vi "main.vi"() -> ()   [LabVIEW 2016]
uses:
  <vilib>/Instr/_visa.llb/VISA Configure Serial Port (Instr).vi
panel:
  out "强度图":dbl[][](graph)
  out "judge":i32=1
  out "Xloop":dbl
  out "判定":dbl
  out "幅频谱":dbl[](graph)
  out "时域谱":dbl[](graph)
  out "错误输出":errorcluster
  in  "启动":bool
  in  "开始扫描":bool
  in  "X归零":bool
  in  "Y归零":bool
  in  "Y":dbl
  in  "Y轴速度":dbl=3000.0
  in  "X轴速度":dbl=3000.0
  out "电机状态":bool
  out "error out":errorcluster caption="步进电机"
  in  "电机端口":refnum<visa-resource-name>="COM3"
  out "Yloop":dbl
  in  "X扫描范围":dbl
  in  "Y扫描范围":dbl=1.0
  out "Y序":i32
  in  "X":dbl
  out "Y(mm)":dbl
  out "x+y 2":dbl
  in  "Y步进":dbl=1.0
  in  "精度":dbl
  in  "电机急停":bool
  out "X（mm）":dbl
  out "x+y":dbl
  in  "X步进":dbl=1.0
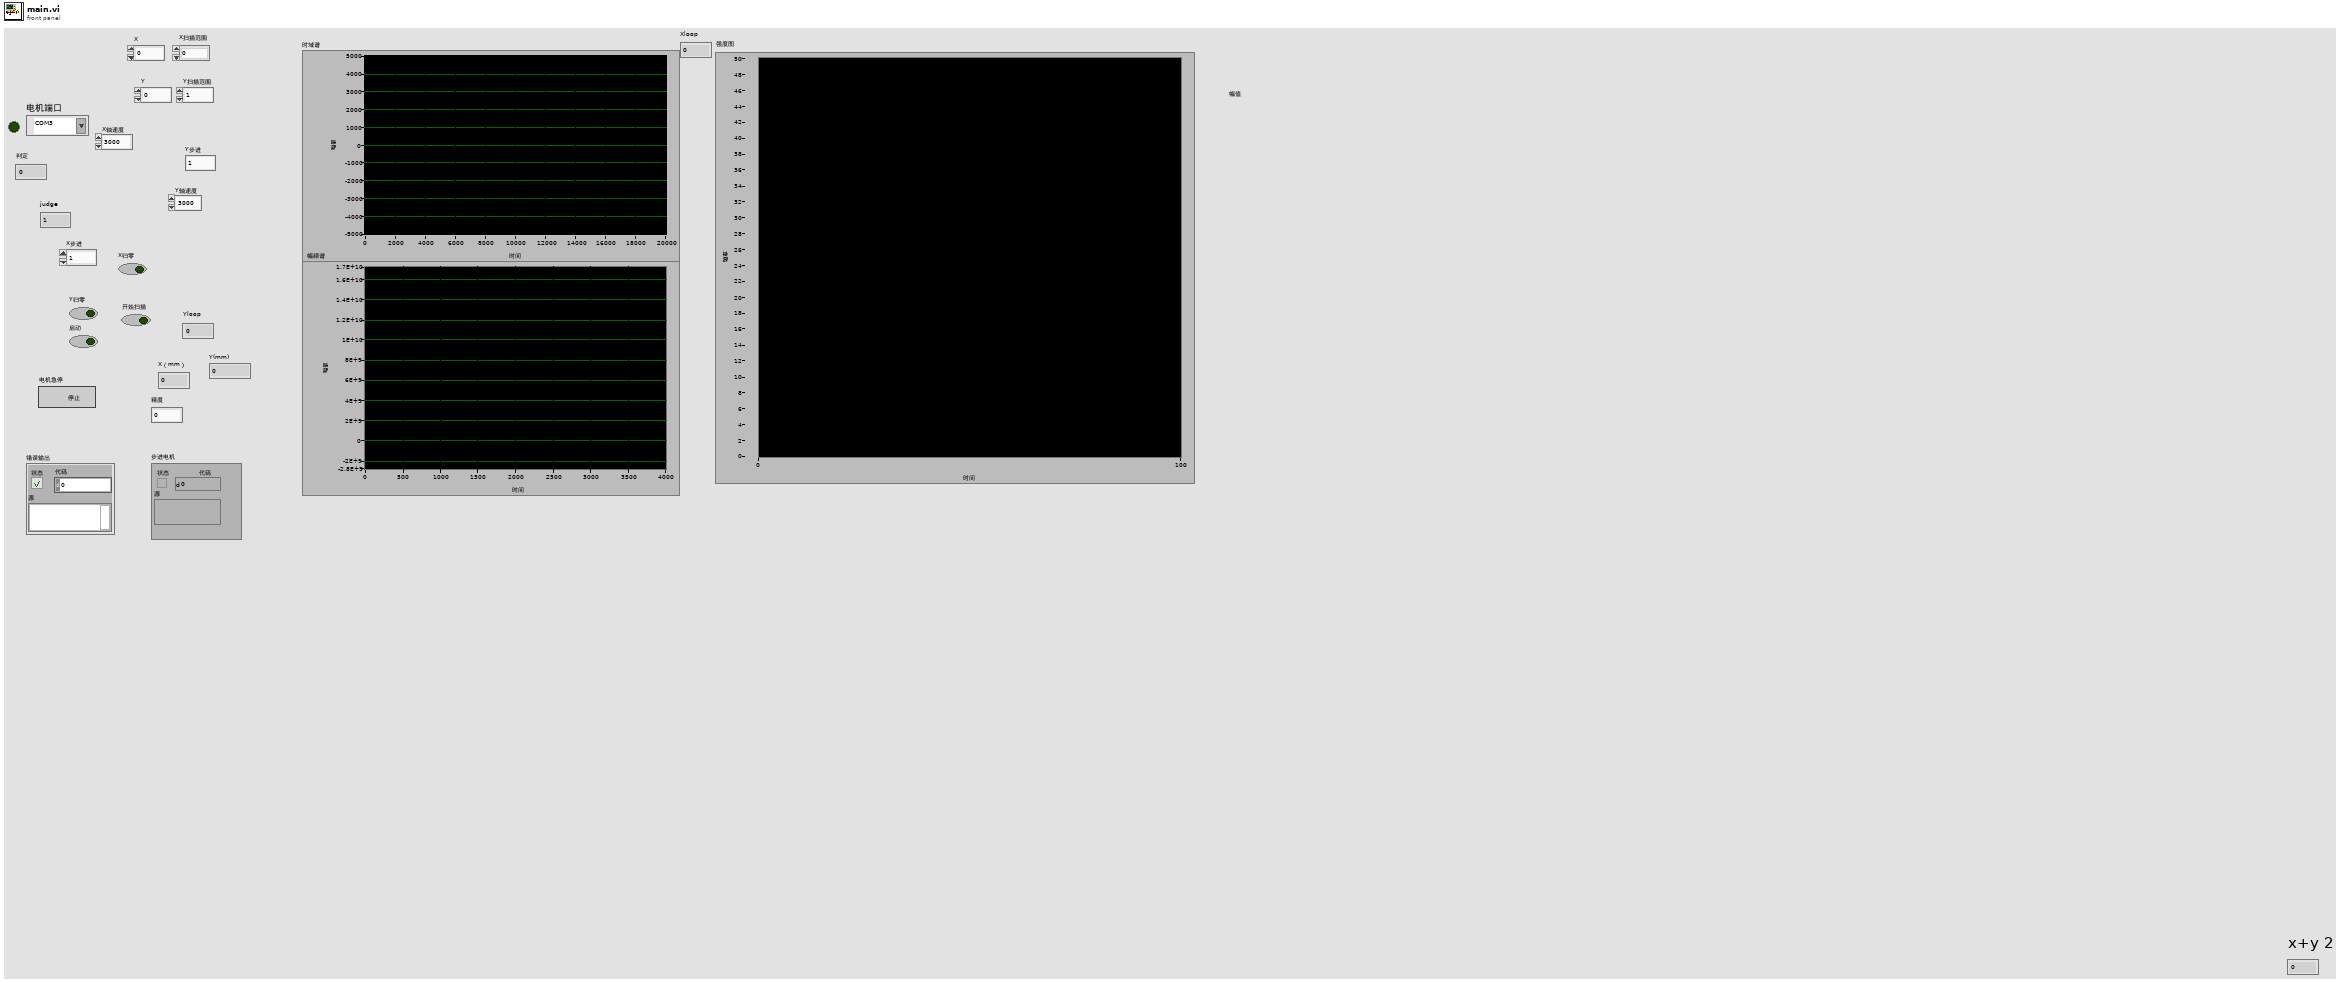
[diagram p1: front panel]
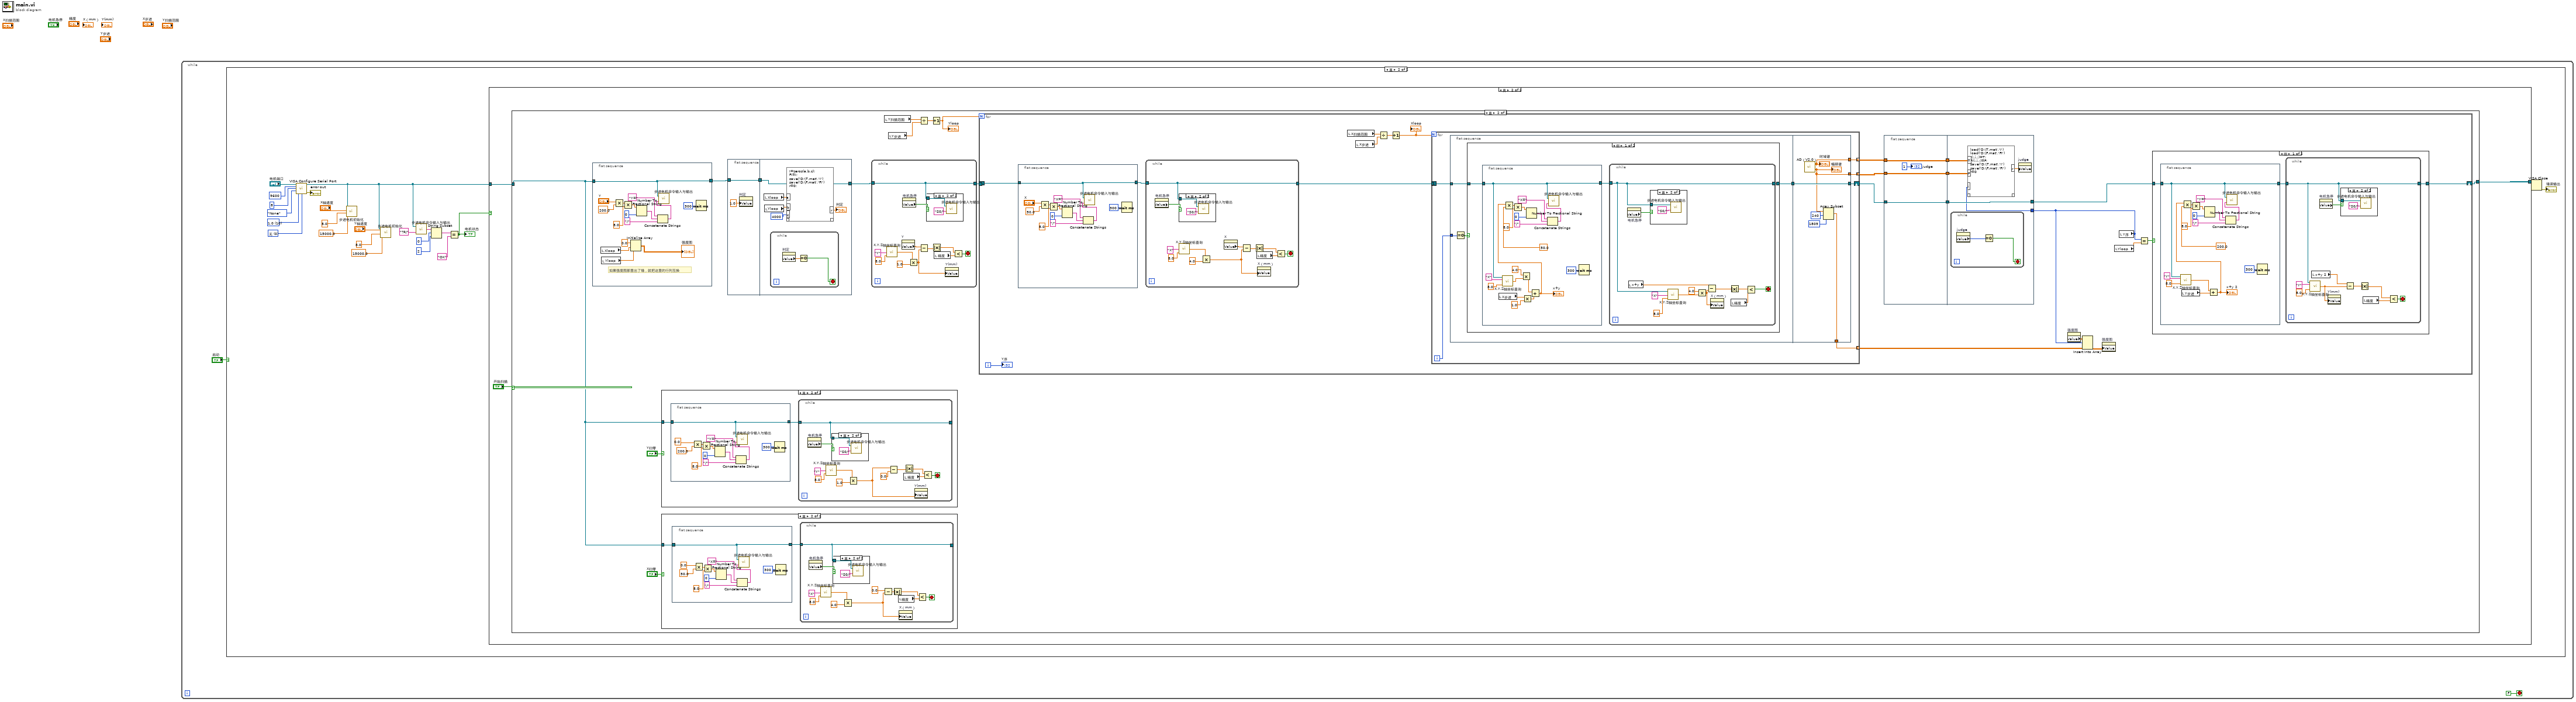
[diagram p0: block diagram]
diagram:
  n1 = while {
    stop <- FALSE stop-if-true
    n2 = case shown="真" "启动" {
      frame False {
      }
      frame True {
        w20 = u16 0 items=["无", "XON/XOFF", "RTS/CTS", "XON/XOFF & RTS/CTS", "DTR/DSR", "XON/XOFF & DTR/DSR"] ("flow control (0:none)")
        w21 = u16 10 items=["1.0"=10, "1.5"=15, "2.0"=20] ("stop bits (10: 1 bit)")
        n3 = call-poly "VISA Configure Serial Port"("VISA resource name"="电机端口", "baud rate (9600)"=u32 9600, "data bits (8)"=u16 8, "parity (0:none)"=enum16{"None", "Odd", "Even", "Mark", "Space"}."None", "stop bits (10: 1 bit)"=w21, "flow control (0:none)"=w20) -> ("VISA resource name out"=w6:refnum<visa-resource-name>, "error out"=→"error out":errorcluster)  [unwired: 1 in, 7 out]
        n4 = call "步进电机初始化.vi"("回零速度"=15000.0, "细分设置"=8.0, "X轴速度"="X轴速度", "串口通信端口"=w6) -> ()  [unwired: 2 in, 1 out]
        n5 = call "步进电机初始化.vi"("Y轴速度"="Y轴速度", "回零速度"=15000.0, "细分设置"=8.0, "串口通信端口"=w6) -> ()  [unwired: 2 in, 1 out]
        n6 = call "步进电机命令输入与输出.vi"("输入字符串"="?R/", "串口通信端口"=w6) -> ("返回字符串"=w16:string)
        n7 = String Subset(string=w16, offset (0)=0 ("偏移量(0)"), length (rest)=2 ("长度（剩余）")) -> (substring=w13:string)
        n8 = Equal?(x=w13, y="OK") -> (x = y?=w5:bool)
        "电机状态" <- w5
        n9 = case shown="真" w5 {
          tunnel: w6 -> [w26 w29]
          tunnel: [w26 w27] -> w4
          frame False {
          }
          frame True {
            n10 = case shown="真" "开始扫描" {
              tunnel: w29 -> [w30 w41]
              tunnel: [w30 w34] -> w27
              frame False {
              }
              frame True {
                n11 = flat-sequence {
                  tunnel: w41 -> [w57]
                  tunnel: [w57] -> w33
                  frame #0 {
                    # "如果强度图那里出了错，就把这里的行列互换"
                    n12 = local read "Xloop"() -> (w54:dbl)
                    n13 = local read "Yloop"() -> (w53:dbl)
                    n14 = Multiply(x="Y", y=200.0) -> (x*y=w62:dbl)
                    n15 = Multiply(x=w62, y=8.0 ("细分设置")) -> (x*y=w67:dbl)
                    n16 = Initialize Array(0.0 ("元素"), w54, w53) -> (→"强度图":dbl[][])
                    n17 = Number To Fractional String(number=w67, precision (6)=i16 0 ("精度(6)")) -> (F-format string=w65:string)  [unwired: 2 out]
                    n18 = Concatenate Strings("Y=" ("字符串"), w65, "/" ("字符串")) -> (w60:string)
                    n19 = call "步进电机命令输入与输出.vi"("输入字符串"=w60, "串口通信端口"=w57) -> ()  [unwired: 1 out]
                    n20 = Wait (ms)(milliseconds to wait=u32 300 ("等待时间（毫秒）")) -> ()  [unwired: 1 out]
                  }
                }
                n21 = case shown="真" "Y归零" {
                  tunnel: w41 -> [_ w110]
                  frame False {
                  }
                  frame True {
                    n22 = flat-sequence {
                      tunnel: w110 -> [w113]
                      tunnel: [w113] -> w111
                      frame #0 {
                        n23 = Multiply(x=0.0, y=200.0) -> (x*y=w118:dbl)
                        n24 = Multiply(x=w118, y=8.0 ("细分设置")) -> (x*y=w123:dbl)
                        n25 = Number To Fractional String(number=w123, precision (6)=i16 0 ("精度(6)")) -> (F-format string=w121:string)  [unwired: 2 out]
                        n26 = Concatenate Strings("Y=" ("字符串"), w121, "/" ("字符串")) -> (w116:string)
                        n27 = call "步进电机命令输入与输出.vi"("输入字符串"=w116, "串口通信端口"=w113) -> ()  [unwired: 1 out]
                        n28 = Wait (ms)(milliseconds to wait=u32 300 ("等待时间（毫秒）")) -> ()  [unwired: 1 out]
                      }
                    }
                    n29 = while {
                      tunnel: [w134] -> _
                      tunnel: w111 -> [w134]
                      stop <- w129 stop-if-true
                      n30 = property on="电机急停" class="Bool (严格)"() -> ("Value"=w130:bool)  [unwired: 2 in, 2 out]
                      n31 = call "X,Y,Z轴坐标查询.vi"("细分设置"=8.0, "查询坐标轴"="Y") -> ("坐标(mm)"=w131:dbl)  [unwired: 1 in]
                      n32 = case shown="真" w130 {
                        tunnel: w134 -> [_ w136]
                        frame False {
                        }
                        frame True {
                          n33 = call "步进电机命令输入与输出.vi"("输入字符串"="S0/", "串口通信端口"=w136) -> ()  [unwired: 1 out]
                        }
                      }
                      n34 = Multiply(x=w131, y=1.0 ("x")) -> (x*y=w127:dbl)
                      n35 = Subtract(x=w127, y=0.0 ("x")) -> (x-y=w125:dbl)
                      n36 = local read "精度"() -> (w128:dbl)
                      n37 = Absolute Value(x=w125) -> (abs(x)=w124:dbl)
                      n38 = property on="Y(mm)" class="DigNum (严格)"("Value"=w127) -> ()  [unwired: 2 in, 2 out]
                      n39 = Less?(x=w124, y=w128) -> (x < y?=w129:bool)
                    }
                  }
                }
                n40 = case shown="真" "X归零" {
                  tunnel: w41 -> [_ w82]
                  frame False {
                  }
                  frame True {
                    n41 = flat-sequence {
                      tunnel: w82 -> [w85]
                      tunnel: [w85] -> w83
                      frame #0 {
                        n42 = Multiply(x=0.0, y=50.0) -> (x*y=w90:dbl)
                        n43 = Multiply(x=w90, y=8.0 ("细分设置")) -> (x*y=w95:dbl)
                        n44 = Number To Fractional String(number=w95, precision (6)=i16 0 ("精度(6)")) -> (F-format string=w93:string)  [unwired: 2 out]
                        n45 = Concatenate Strings("X=" ("字符串"), w93, "/" ("字符串")) -> (w88:string)
                        n46 = call "步进电机命令输入与输出.vi"("输入字符串"=w88, "串口通信端口"=w85) -> ()  [unwired: 1 out]
                        n47 = Wait (ms)(milliseconds to wait=u32 300 ("等待时间（毫秒）")) -> ()  [unwired: 1 out]
                      }
                    }
                    n48 = while {
                      tunnel: [w106] -> _
                      tunnel: w83 -> [w106]
                      stop <- w101 stop-if-true
                      n49 = property on="电机急停" class="Bool (严格)"() -> ("Value"=w102:bool)  [unwired: 2 in, 2 out]
                      n50 = call "X,Y,Z轴坐标查询.vi"("细分设置"=8.0, "查询坐标轴"="X") -> ("坐标(mm)"=w103:dbl)  [unwired: 1 in]
                      n51 = case shown="真" w102 {
                        tunnel: w106 -> [_ w108]
                        frame False {
                        }
                        frame True {
                          n52 = call "步进电机命令输入与输出.vi"("输入字符串"="S0/", "串口通信端口"=w108) -> ()  [unwired: 1 out]
                        }
                      }
                      n53 = Multiply(x=w103, y=4.0 ("x")) -> (x*y=w99:dbl)
                      n54 = Subtract(x=0.0, y=w99) -> (x-y=w98:dbl)
                      n55 = Absolute Value(x=w98) -> (abs(x)=w97:dbl)
                      n56 = local read "精度"() -> (w100:dbl)
                      n57 = property on="X（mm）" class="DigNum (严格)"("Value"=w99) -> ()  [unwired: 2 in, 2 out]
                      n58 = Less?(x=w97, y=w100) -> (x < y?=w101:bool)
                    }
                  }
                }
                n59 = flat-sequence {
                  tunnel: w33 -> [w43]
                  tunnel: [w43] -> w32
                  tunnel: [w45] -> _
                  tunnel: w32 -> [w45]
                  tunnel: [w45] -> w31
                  frame #0 {
                    n60 = property on="判定" class="DigNum (严格)"("Value"=1.0 ("判定")) -> ()  [unwired: 2 in, 2 out]
                  }
                  frame #1 {
                    n61 = local read "Xloop"() -> (w48:dbl)
                    n62 = local read "Yloop"() -> (w47:dbl)
                    n63 = while {
                      stop <- w50 stop-if-true
                      n64 = property on="判定" class="DigNum (严格)"() -> ("Value"=w51:dbl)  [unwired: 2 in, 2 out]
                      n65 = Equal To 0?(x=w51) -> (x = 0?=w50:bool)
                    }
                    n66 = script code="I=zeros(a,b,c);\nFI=I;\nsave('D:\\T.mat','I') \nsave('D:\\F.mat','FI') \nr=0;"("a"=w48, "b"=w47, "c"=4000) -> ("r"=→"判定":dbl)  [unwired: 1 in, 1 out]
                  }
                }
                n67 = while {
                  tunnel: [w78] -> w42
                  tunnel: w31 -> [w78]
                  stop <- w72 stop-if-true
                  n68 = call "X,Y,Z轴坐标查询.vi"("细分设置"=8.0, "查询坐标轴"="Y") -> ("坐标(mm)"=w74:dbl)  [unwired: 1 in]
                  n69 = property on="Y" class="DigNum (严格)"() -> ("Value"=w76:dbl)  [unwired: 2 in, 2 out]
                  n70 = property on="电机急停" class="Bool (严格)"() -> ("Value"=w73:bool)  [unwired: 2 in, 2 out]
                  n71 = Multiply(x=w74, y=1.0 ("x")) -> (x*y=w70:dbl)
                  n72 = Subtract(x=w76, y=w70) -> (x-y=w69:dbl)
                  n73 = case shown="真" w73 {
                    tunnel: w78 -> [_ w80]
                    frame False {
                    }
                    frame True {
                      n74 = call "步进电机命令输入与输出.vi"("输入字符串"="S0/", "串口通信端口"=w80) -> ()  [unwired: 1 out]
                    }
                  }
                  n75 = Absolute Value(x=w69) -> (abs(x)=w68:dbl)
                  n76 = local read "精度"() -> (w71:dbl)
                  n77 = property on="Y(mm)" class="DigNum (严格)"("Value"=w70) -> ()  [unwired: 2 in, 2 out]
                  n78 = Less?(x=w68, y=w71) -> (x < y?=w72:bool)
                }
                n79 = local read "Y扫描范围"() -> (w37:dbl)
                n80 = local read "Y步进"() -> (w38:dbl)
                n81 = Divide(x=w37, y=w38) -> (x/y=w36:dbl)
                n82 = Increment(x=w36) -> (x+1=w35:dbl)
                "Yloop" <- w35
                n83 = for {
                  N: w35 -> [_]
                  tunnel: w42 -> [w151]
                  shift-right: [w150] -> w34
                  shift-left: _ -> [_]
                  i -> [w157]
                  n84 = flat-sequence {
                    tunnel: w151 -> [w172]
                    tunnel: [w172] -> w149
                    frame #0 {
                      n85 = Multiply(x="X", y=50.0) -> (x*y=w177:dbl)
                      n86 = Multiply(x=w177, y=8.0 ("细分设置")) -> (x*y=w182:dbl)
                      n87 = Number To Fractional String(number=w182, precision (6)=i16 0 ("精度(6)")) -> (F-format string=w180:string)  [unwired: 2 out]
                      n88 = Concatenate Strings("X=" ("字符串"), w180, "/" ("字符串")) -> (w175:string)
                      n89 = call "步进电机命令输入与输出.vi"("输入字符串"=w175, "串口通信端口"=w172) -> ()  [unwired: 1 out]
                      n90 = Wait (ms)(milliseconds to wait=u32 300 ("等待时间（毫秒）")) -> ()  [unwired: 1 out]
                    }
                  }
                  n91 = while {
                    tunnel: [w193] -> w158
                    tunnel: w149 -> [w193]
                    stop <- w187 stop-if-true
                    n92 = property on="电机急停" class="Bool (严格)"() -> ("Value"=w188:bool)  [unwired: 2 in, 2 out]
                    n93 = case shown="真" w188 {
                      tunnel: w193 -> [_ w195]
                      frame False {
                      }
                      frame True {
                        n94 = call "步进电机命令输入与输出.vi"("输入字符串"="S0/", "串口通信端口"=w195) -> ()  [unwired: 1 out]
                      }
                    }
                    n95 = call "X,Y,Z轴坐标查询.vi"("细分设置"=8.0, "查询坐标轴"="X") -> ("坐标(mm)"=w189:dbl)  [unwired: 1 in]
                    n96 = Multiply(x=w189, y=4.0 ("x")) -> (x*y=w185:dbl)
                    n97 = property on="X" class="DigNum (严格)"() -> ("Value"=w191:dbl)  [unwired: 2 in, 2 out]
                    n98 = Subtract(x=w191, y=w185) -> (x-y=w184:dbl)
                    n99 = Absolute Value(x=w184) -> (abs(x)=w183:dbl)
                    n100 = local read "精度"() -> (w186:dbl)
                    n101 = property on="X（mm）" class="DigNum (严格)"("Value"=w185) -> ()  [unwired: 2 in, 2 out]
                    n102 = Less?(x=w183, y=w186) -> (x < y?=w187:bool)
                  }
                  n103 = local read "X扫描范围"() -> (w153:dbl)
                  n104 = local read "X步进"() -> (w152:dbl)
                  n105 = Divide(x=w153, y=w152) -> (x/y=w155:dbl)
                  n106 = Increment(x=w155) -> (x+1=w154:dbl)
                  "Xloop" <- w154
                  n107 = for {
                    N: w154 -> [_]
                    tunnel: w158 -> [w234]
                    shift-right: [w232] -> w144
                    shift-left: _ -> [_]
                    tunnel: [w231] -> w148 mode=indexing
                    tunnel: [w230] -> w147 mode=indexing
                    tunnel: [w229] -> w138 mode=indexing
                    i -> [w235]
                    n108 = flat-sequence {
                      tunnel: w235 -> [w238]
                      tunnel: w234 -> [w237]
                      tunnel: [w236] -> w233
                      tunnel: [w283] -> w232
                      tunnel: w233 -> [w283]
                      tunnel: [w282] -> w231
                      tunnel: [w281] -> w230
                      tunnel: [w278] -> w229
                      frame #0 {
                        n109 = Equal To 0?(x=w238) -> (x = 0?=w239:bool)
                        n110 = case shown="假" w239 {
                          tunnel: w237 -> [w241 w277]
                          tunnel: [w240 w277] -> w236
                          frame False {
                            n111 = flat-sequence {
                              tunnel: w241 -> [w249]
                              tunnel: [w249] -> w242
                              frame #0 {
                                n112 = local read "X步进"() -> (w243:dbl)
                                n113 = call "X,Y,Z轴坐标查询.vi"("细分设置"=8.0, "查询坐标轴"="X", "串口通信端口"=w249) -> ("坐标(mm)"=w245:dbl)
                                n114 = Multiply(x=4.0, y=w245) -> (x*y=w244:dbl)
                                n115 = Multiply(x=w243, y=1.0 ("x")) -> (x*y=w248:dbl)
                                n116 = Add(x=w244, y=w248) -> (x+y=w252:dbl)
                                "x+y" <- w252
                                n117 = Multiply(x=w252, y=50.0) -> (x*y=w257:dbl)
                                n118 = Multiply(x=w257, y=8.0 ("细分设置")) -> (x*y=w262:dbl)
                                n119 = Number To Fractional String(number=w262, precision (6)=i16 0 ("精度(6)")) -> (F-format string=w260:string)  [unwired: 2 out]
                                n120 = Concatenate Strings("X=" ("字符串"), w260, "/" ("字符串")) -> (w255:string)
                                n121 = call "步进电机命令输入与输出.vi"("输入字符串"=w255, "串口通信端口"=w249) -> ()  [unwired: 1 out]
                                n122 = Wait (ms)(milliseconds to wait=u32 300 ("等待时间（毫秒）")) -> ()  [unwired: 1 out]
                              }
                            }
                            n123 = while {
                              tunnel: [w272] -> w240
                              tunnel: w242 -> [w272]
                              stop <- w271 stop-if-true
                              n124 = property on="电机急停" class="Bool (严格)"() -> ("Value"=w268:bool)  [unwired: 2 in, 2 out]
                              n125 = local read "x+y"() -> (w273:dbl)
                              n126 = case shown="真" w268 {
                                tunnel: w272 -> [_ w275]
                                frame False {
                                }
                                frame True {
                                n127 = call "步进电机命令输入与输出.vi"("输入字符串"="S0/", "串口通信端口"=w275) -> ()  [unwired: 1 out]
                                }
                              }
                              n128 = call "X,Y,Z轴坐标查询.vi"("细分设置"=8.0, "查询坐标轴"="X", "串口通信端口"=w272) -> ("坐标(mm)"=w266:dbl)
                              n129 = Multiply(x=4.0, y=w266) -> (x*y=w265:dbl)
                              n130 = Subtract(x=w273, y=w265) -> (x-y=w264:dbl)
                              n131 = property on="X（mm）" class="DigNum (严格)"("Value"=w265) -> ()  [unwired: 2 in, 2 out]
                              n132 = Absolute Value(x=w264) -> (abs(x)=w263:dbl)
                              n133 = local read "精度"() -> (w267:dbl)
                              n134 = Less?(x=w263, y=w267) -> (x < y?=w271:bool)
                            }
                          }
                          frame True {
                          }
                        }
                      }
                      frame #1 {
                        n135 = call "AD（V2.0）.vi"() -> ("时域谱"=w282:dbl[], "幅频谱"=w281:dbl[])  [unwired: 1 in]
                        "时域谱" <- w282
                        "幅频谱" <- w281
                        n136 = Array Subset(array=w281, index=240 ("索引"), length=1809 ("长度")) -> (w278:dbl[])
                      }
                    }
                  }
                  n137 = flat-sequence {
                    tunnel: w147 -> [w162]
                    tunnel: w148 -> [w163]
                    tunnel: [w163] -> w146
                    tunnel: [w162] -> w145
                    tunnel: w144 -> [w160]
                    tunnel: [w160] -> w143
                    tunnel: w146 -> [w168]
                    tunnel: w145 -> [w167]
                    tunnel: w143 -> [w165]
                    tunnel: [w165] -> w142
                    tunnel: w139 -> [w164]
                    frame #0 {
                      "judge" <- 1
                    }
                    frame #1 {
                      n138 = while {
                        stop <- w170 stop-if-true
                        n139 = property on="judge" class="DigNum (严格)"() -> ("Value"=w169:i32)  [unwired: 2 in, 2 out]
                        n140 = Equal To 0?(x=w169) -> (x = 0?=w170:bool)
                      }
                      n141 = script code="load('D:\\T.mat','I') \nload('D:\\F.mat','FI') \nI(:,i,:)=T;\nFI(:,i,:)=F;\nsave('D:\\T.mat','I') \nsave('D:\\F.mat','FI') \nr=0"("i"=w164, "T"=w168, "F"=w167) -> ("r"=w166:dbl)  [unwired: 1 in, 1 out]
                      n142 = property on="judge" class="DigNum (严格)"("Value"=w166) -> ()  [unwired: 2 in, 2 out]
                    }
                  }
                  n143 = property on="强度图" class="IntGraph (严格)"() -> ("Value"=w140:dbl[][])  [unwired: 2 in, 2 out]
                  n144 = local read "Yloop"() -> (w156:dbl)
                  n145 = local read "Y序"() -> (w139:i32)
                  n146 = Insert Into Array(array=w140, index (row)=w139, new element=w138) -> (w141:dbl[][])  [unwired: 1 in]
                  n147 = property on="强度图" class="IntGraph (严格)"("Value"=w141) -> ()  [unwired: 2 in, 2 out]
                  n148 = Equal?(x=w139, y=w156) -> (x = y?=w159:bool)
                  n149 = case shown="假" w159 {
                    tunnel: w142 -> [w199 w228]
                    tunnel: [w197 w228] -> w150
                    frame False {
                      n150 = flat-sequence {
                        tunnel: w199 -> [w200]
                        tunnel: [w200] -> w198
                        frame #0 {
                          n151 = call "X,Y,Z轴坐标查询.vi"("细分设置"=8.0, "查询坐标轴"="Y", "串口通信端口"=w200) -> ("坐标(mm)"=w202:dbl)
                          n152 = local read "Y步进"() -> (w201:dbl)
                          n153 = Add(x=w202, y=w201) -> (x+y=w205:dbl)
                          "x+y 2" <- w205
                          n154 = Multiply(x=w205, y=200.0) -> (x*y=w210:dbl)
                          n155 = Multiply(x=w210, y=8.0 ("细分设置")) -> (x*y=w215:dbl)
                          n156 = Number To Fractional String(number=w215, precision (6)=i16 0 ("精度(6)")) -> (F-format string=w213:string)  [unwired: 2 out]
                          n157 = Concatenate Strings("Y=" ("字符串"), w213, "/" ("字符串")) -> (w208:string)
                          n158 = call "步进电机命令输入与输出.vi"("输入字符串"=w208, "串口通信端口"=w200) -> ()  [unwired: 1 out]
                          n159 = Wait (ms)(milliseconds to wait=u32 300 ("等待时间（毫秒）")) -> ()  [unwired: 1 out]
                        }
                      }
                      n160 = while {
                        tunnel: [w216] -> w197
                        tunnel: w198 -> [w216]
                        stop <- w223 stop-if-true
                        n161 = call "X,Y,Z轴坐标查询.vi"("细分设置"=8.0, "查询坐标轴"="Y", "串口通信端口"=w216) -> ("坐标(mm)"=w220:dbl)
                        n162 = local read "x+y 2"() -> (w224:dbl)
                        n163 = property on="电机急停" class="Bool (严格)"() -> ("Value"=w219:bool)  [unwired: 2 in, 2 out]
                        n164 = property on="Y(mm)" class="DigNum (严格)"("Value"=w220) -> ()  [unwired: 2 in, 2 out]
                        n165 = case shown="真" w219 {
                          tunnel: w216 -> [_ w226]
                          frame False {
                          }
                          frame True {
                            n166 = call "步进电机命令输入与输出.vi"("输入字符串"="S0/", "串口通信端口"=w226) -> ()  [unwired: 1 out]
                          }
                        }
                        n167 = Subtract(x=w224, y=w220) -> (x-y=w218:dbl)
                        n168 = Absolute Value(x=w218) -> (abs(x)=w217:dbl)
                        n169 = local read "精度"() -> (w221:dbl)
                        n170 = Less?(x=w217, y=w221) -> (x < y?=w223:bool)
                      }
                    }
                    frame True {
                    }
                  }
                  "Y序" <- w157
                }
              }
            }
          }
        }
        n171 = VISA Close(VISA resource name=w4) -> (error out=→"错误输出":errorcluster)  [unwired: 1 in]
      }
    }
  }
